vi "Read.vi"() -> ()   [LabVIEW 2020]
panel:
  in  "Tab Control":enum32{"Data", "Error"}(tab)
  out "Thermometer":dbl(slide) scale=0.0..100.0
  in  "stop":bool
  in  "PORT":u16
  out "error out":errorcluster
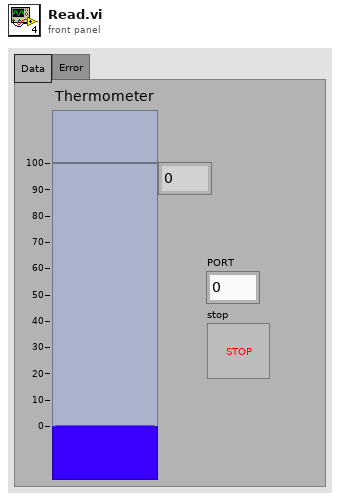
[diagram p1: front panel]
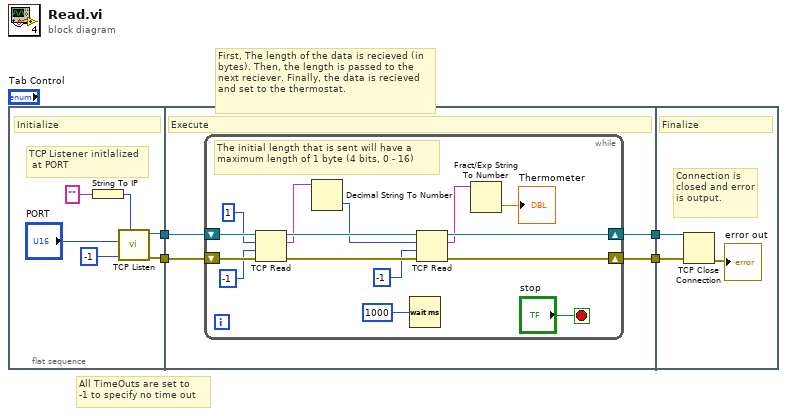
[diagram p0: block diagram]
diagram:
  # "First, The length of the data is recieved (in bytes). Then, the length is passed to the next reciever. Finally, the data is recieved and set to the thermostat."
  # "All TimeOuts are set to \n-1 to specify no time out"
  n1 = flat-sequence {
    tunnel: [w7] -> w4
    tunnel: [w8] -> w3
    tunnel: w4 -> [w14]
    tunnel: w3 -> [w12]
    tunnel: [w13] -> w2
    tunnel: [w11] -> w1
    tunnel: w2 -> [w31]
    tunnel: w1 -> [w32]
    frame #0 {
      # "TCP Listener initlalized\n at PORT"
      # "Initialize"
      n2 = String To IP(1:"" ("name")) -> (0:w5:u32)
      n3 = call <vilib>:"TCP Listen.vi"("net address"=w5, "timeout ms (wait forever: -1)"=-1, "port"="PORT") -> ("error out"=w8:errorcluster, "connection ID"=w7:refnum<k5>)  [unwired: 4 in, 3 out]
    }
    frame #1 {
      # "Execute"
      n4 = while {
        shift-right: [w27] -> w13
        shift-left: w14 -> [w29]
        shift-right: [w24] -> w11
        shift-left: w12 -> [w26]
        stop <- "stop" stop-if-true
        # "The initial length that is sent will have a maximum length of 1 byte (4 bits, 0 - 16)"
        n5 = TCP Read(connection ID=w29, bytes to read=1, error in (no error)=w26, 9:-1 ("timeout ms (25000)")) -> (connection ID out=w28:refnum<k5>, data out=w21:string, error out=w25:errorcluster)  [unwired: 1 in]
        n6 = Decimal String To Number(string=w21) -> (number=w20:i32)  [unwired: 2 in, 1 out]
        n7 = Wait (ms)(milliseconds to wait=u32 1000) -> ()  [unwired: 1 out]
        n8 = TCP Read(connection ID=w28, bytes to read=w20, error in (no error)=w25, 9:-1 ("timeout ms (25000)")) -> (connection ID out=w27:refnum<k5>, data out=w23:string, error out=w24:errorcluster)  [unwired: 1 in]
        n9 = Fract/Exp String To Number(string=w23) -> (number=→"Thermometer":dbl)  [unwired: 3 in, 1 out]
      }
    }
    frame #2 {
      # "Connection is closed and error is output."
      # "Finalize"
      n10 = TCP Close Connection(connection ID=w31, error in (no error)=w32) -> (error out=→"error out":errorcluster)  [unwired: 1 in, 1 out]
    }
  }
